vi "OffsetRect by Point and Rect Array.vi"(8 "错误输入":errorcluster, 10 "point":cluster{"x":i16, "y":i16} caption="点", 11 "Rect Array":T1(array[cluster])) -> (0 "错误输出":errorcluster, 3 "OffsetRect Array":T1(array[cluster]))   [LabVIEW 2012, in "Picture Box Tools.lvlib" / "Rect Tools.lvlib"]
uses:
  Rect Tools.lvlib
  OffsetRect by Point and Rect.vi
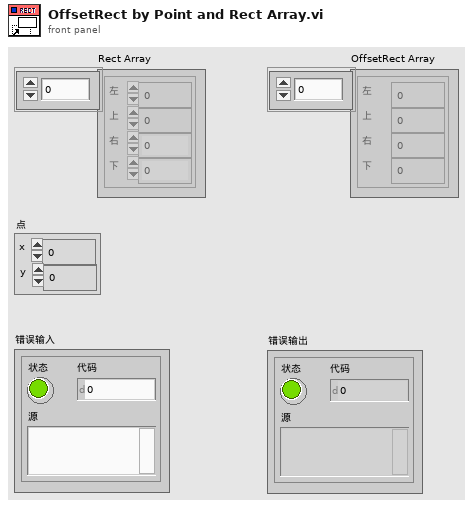
[diagram p1: front panel]
types:
  T1 = cluster{"left":i16, "top":i16, "right":i16, "bottom":i16}[]
  T2 = cluster{"left":i16, "top":i16, "right":i16, "bottom":i16}
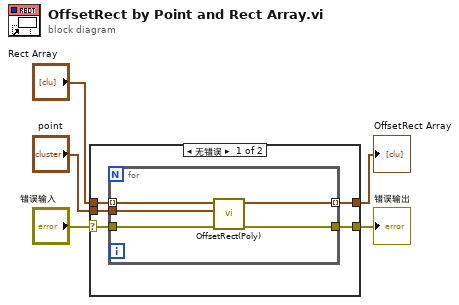
[diagram p0: block diagram]
diagram:
  n1 = case shown="无错误" "错误输入" {
    selector: "错误输入" -> [w8 w17]
    tunnel: [w7 w17] -> w1
    tunnel: "point" -> [w9 _]
    tunnel: "Rect Array" -> [w10 w16]
    tunnel: [w6 w16] -> w2
    frame No Error {
      n2 = for {
        tunnel: w10 -> [w15] mode=indexing
        tunnel: w9 -> [w14]
        tunnel: w8 -> [w13]
        tunnel: [w12] -> w7
        tunnel: [w11] -> w6 mode=indexing
        n3 = call-poly "OffsetRect(Poly).vi"("错误输入"=w13, "point"=w14, "rect"=w15) -> ("错误输出"=w12:errorcluster, "offset rect"=w11:T2)  [unwired: 7 in]
      }
    }
    frame Error {
    }
  }
  "错误输出" <- w1
  "OffsetRect Array" <- w2
